vi "FPGA_drive_steering.vi"() -> ()   [LabVIEW 2019]
uses:
  <vilib>/rvi/Emulation/niFpgaGetClockAttributes.vi
  <vilib>/rvi/Emulation/niFpgaSctlEmulationGetInTimedLoop.vi
  <vilib>/rvi/Emulation/niFpgaEmulationReportErrorSimple.vi
  <vilib>/rvi/Emulation/niFpgaCriticalErrorInLSC.vi
  Sub VIs/Drive/UART 8N1/UART 8N1 (FPGA).lvlib
panel:
  in  "Frequency (Hz)":sgl
  in  "Duty Cycle (%)":sgl
  in  "Baud Rate":u32=9600
  in  "Write Data":u8[](array[numeric])=[0, 0, 0, 0, 0, 0, 0, 0, 0, 0, 0, 0, 0, 0, 0, 0, 0, 0, 0, 0, 0, 0, 0, 0, 0, 0, 0, 0, 0, 0, 0, 0, 0, 0, 0, 0, 0, 0, 0, 0, 0, 0, 0, 0, 0, 0, 0, 0, 0, 0]
  in  "Write":bool
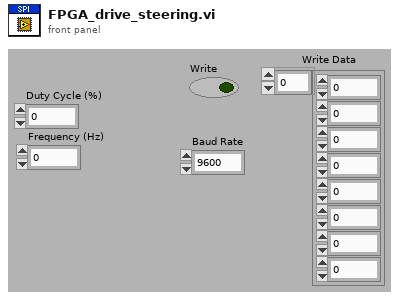
[diagram p1: front panel]
types:
  T1 = typedef "UART 8N1 (FPGA).lvlib/UART Ref.ctl" = cluster{"FPGA I/O":refnum<k21>, "Buffer Ref":refnum<k21>, "Stop Ref":refnum<k21>}
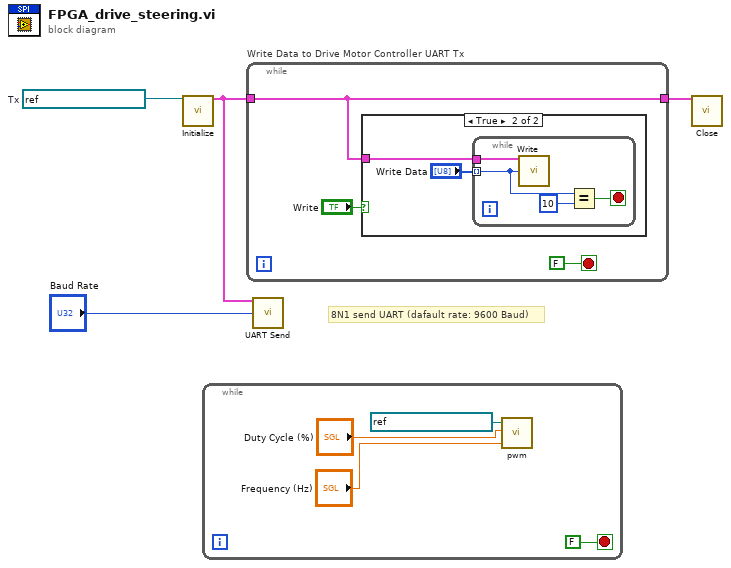
[diagram p0: block diagram]
diagram:
  w4 = refnum<k21> "ConnectorA/DIO1"  # Tx
  # "8N1 send UART (dafault rate: 9600 Baud)"
  n1 = call "Initialize.vi"("FPGA I/O"=w4) -> ("BPT Ref"=w3:T1)  [unwired: 14 in]
  n2 = while {
    stop <- FALSE stop-if-true
    n3 = call "pwm.vi"("Frequency (Hz)"="Frequency (Hz)", "Duty Cycle (%)"="Duty Cycle (%)", "FPGA I/O In"=refnum<k21> "ConnectorB/DIO1") -> ()  [unwired: 1 in]
  }
  n4 = while "Write Data to Drive Motor Controller UART Tx" {
    tunnel: w3 -> [w10]
    tunnel: [w10] -> w2
    stop <- FALSE stop-if-true
    n5 = case "Write" shown="True" "Write" {
      tunnel: w10 -> [_ w13]
      frame False {
      }
      frame True {
        n6 = while {
          tunnel: w13 -> [w17]
          tunnel: "Write Data" -> [w15] mode=indexing
          stop <- w16 stop-if-true
          n7 = call "Write.vi"("UART Ref In"=w17, "Data"=w15) -> ()  [unwired: 12 in, 2 out]
          n8 = Equal?(x=w15, y=u8 10) -> (x = y?=w16:bool)
        }
      }
    }
  }
  n9 = call "UART Send.vi"("UART Ref In"=w3, "Baud Rate (9600)"="Baud Rate") -> ()  [unwired: 14 in]
  n10 = call "Close.vi"("UART Ref"=w2) -> ()  [unwired: 15 in]
